vi "Get Tile ID.vi"(8 "error in (no error)":errorcluster, 11 "Tile in":refnum<class "Tile.lvclass">) -> (0 "error out":errorcluster, 2 "ID":u64, 3 "Tile out":refnum<class "Tile.lvclass">)   [LabVIEW 2020, in "Tile.lvclass"]
uses:
  Tile.lvclass
  Tile.lvclass/Tile.ctl
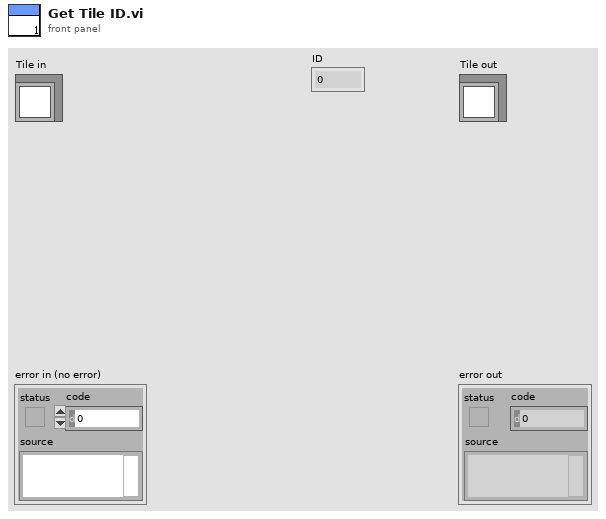
[diagram p1: front panel]
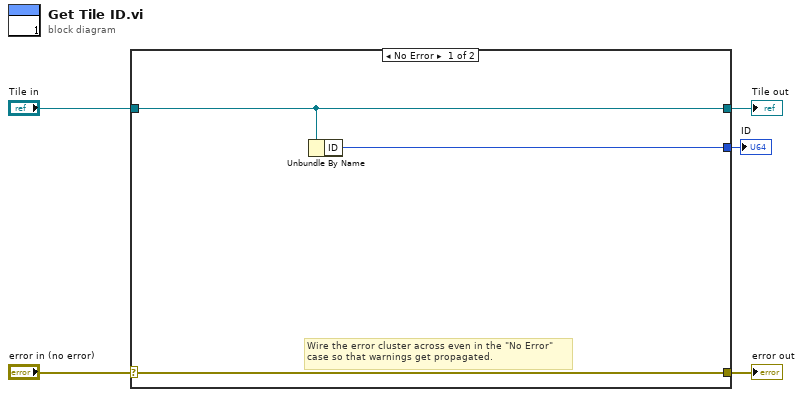
[diagram p0: block diagram]
diagram:
  n1 = case shown="No Error" "error in (no error)" {
    selector: "error in (no error)" -> [w8 w10]
    tunnel: [w8 w10] -> w4
    tunnel: [w7 w9] -> w2
    tunnel: "Tile in" -> [w7 w9]
    tunnel: [w6 _] -> w1
    frame No Error {
      # "Wire the error cluster across even in the \"No Error\"\ncase so that warnings get propagated."
      n2 = Unbundle By Name(w7) -> ("ID"=w6:u64)
    }
    frame Error {
    }
  }
  "error out" <- w4
  "Tile out" <- w2
  "ID" <- w1
